vi "Sub_TaD.vi"() -> ()   [LabVIEW 2020]
panel:
  out "Actual\ntime":string
  in  "STOP":bool
  in  "DATE":bool
  in  "YEAR":i32=2020 min=2010 max=2070 step=1
  in  "MONTH":i32=6 min=1 max=12 step=1
  in  "DAY":i32=15 min=1 max=31 step=1
  in  "TIME":bool
  in  "MINUTE":i32=30 min=-1 max=60 step=1
  in  "HOUR":i32=12 min=-1 max=24 step=1
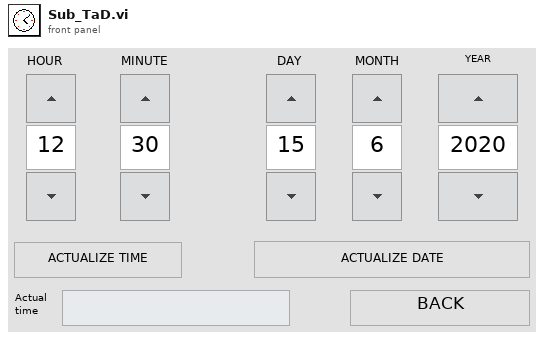
[diagram p1: front panel]
types:
  T1 = enum16{"open", "replace", "create", "open or create", "replace or create", "replace or create with confirmation"}
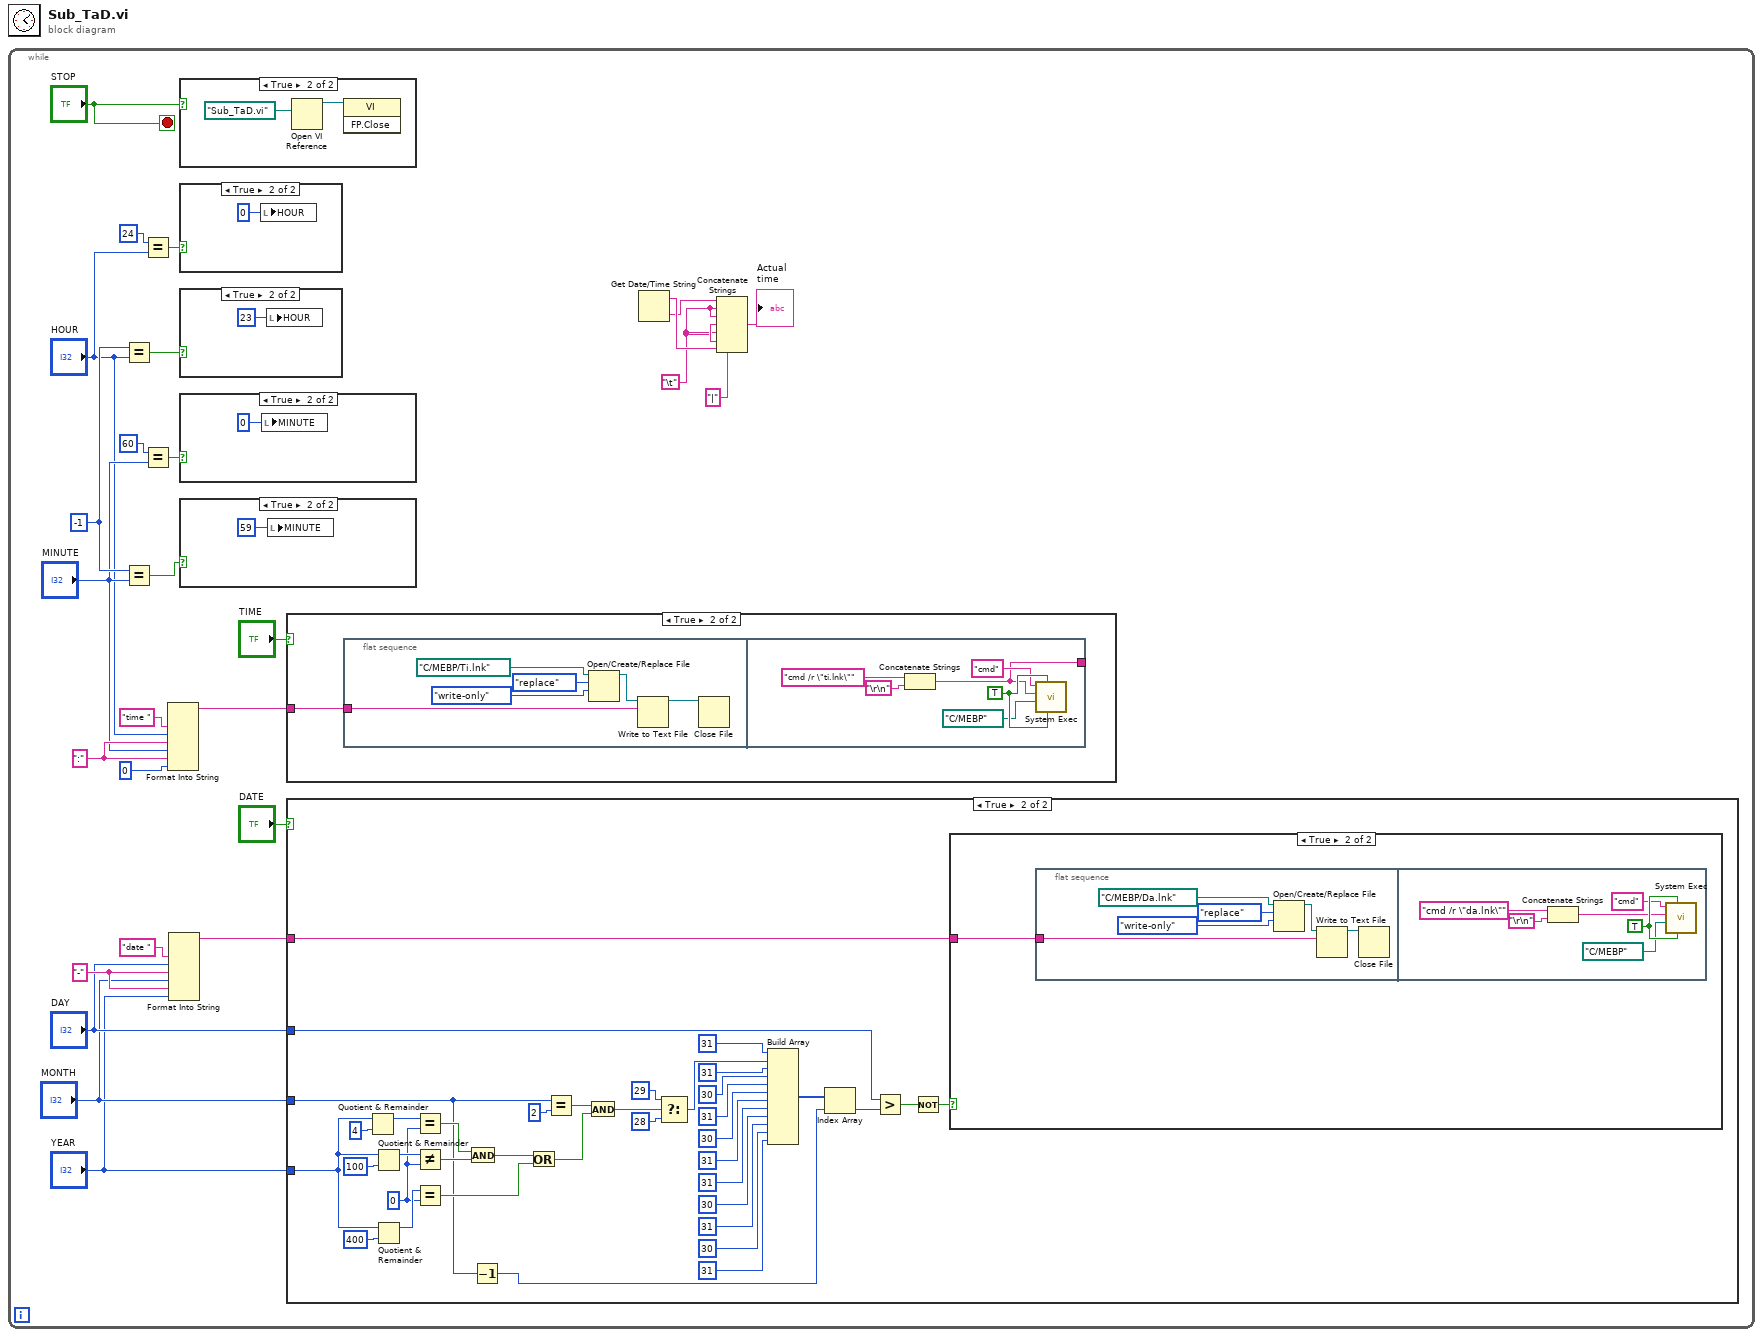
[diagram p0: block diagram]
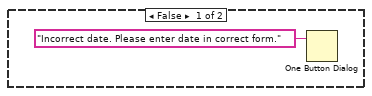
[diagram p4: hidden frame]
diagram:
  n1 = while {
    stop <- "STOP" stop-if-true
    w2 = "\t"
    w13 = "-"
    w24 = -1
    w26 = ":"
    n2 = Equal?(x=w24, y="HOUR") -> (x = y?=w20:bool)
    n3 = Equal?(x=w24, y="MINUTE") -> (x = y?=w19:bool)
    n4 = Equal?(x=24, y="HOUR") -> (x = y?=w21:bool)
    n5 = Equal?(x=60, y="MINUTE") -> (x = y?=w18:bool)
    n6 = Format Into String("time " ("string"), "HOUR", w26, "MINUTE", w26, 0 ("input 6")) -> (resulting string=w11:string)  [unwired: 3 in, 1 out]
    n7 = Format Into String("date " ("string"), "DAY", w13, "MONTH", w13, "YEAR") -> (resulting string=w10:string)  [unwired: 3 in, 1 out]
    n8 = case shown="True" "STOP" {
      frame False {
      }
      frame True {
        n9 = Open VI Reference(vi path=path "Sub_TaD.vi") -> (vi reference=w28:refnum<vi>)  [unwired: 5 in, 1 out]
        n10 = invoke class="VI" method="FP.Close"(reference=w28) -> ()  [unwired: 2 in, 3 out]
      }
    }
    n11 = case shown="True" w21 {
      frame False {
      }
      frame True {
        n12 = local write "HOUR"(0 ("Numeric")) -> ()
      }
    }
    n13 = case shown="True" w20 {
      frame False {
      }
      frame True {
        n14 = local write "HOUR"(23 ("Numeric")) -> ()
      }
    }
    n15 = case shown="True" w18 {
      frame False {
      }
      frame True {
        n16 = local write "MINUTE"(0 ("Numeric 2")) -> ()
      }
    }
    n17 = case shown="True" w19 {
      frame False {
      }
      frame True {
        n18 = local write "MINUTE"(59 ("Numeric 2")) -> ()
      }
    }
    n19 = case shown="True" "TIME" {
      tunnel: w11 -> [_ w82]
      frame False {
      }
      frame True {
        n20 = flat-sequence {
          tunnel: w82 -> [w83]
          tunnel: [w89] -> _
          frame #0 {
            n21 = Open/Create/Replace File(file path (use dialog)=path "C:/MEBP/Ti.lnk", operation (0:open)=T1."replace", access (0:read/write)=enum16{"read/write", "read-only", "write-only"}."write-only") -> (refnum out=w87:refnum<file>)  [unwired: 3 in, 2 out]
            n22 = Write to Text File(file (use dialog)=w87, text=w83) -> (refnum out=w88:refnum<file>)  [unwired: 2 in, 2 out]
            n23 = Close File(refnum=w88) -> ()  [unwired: 1 in, 2 out]
          }
          frame #1 {
            w94 = TRUE ("wait until completion? (T)")
            n24 = Concatenate Strings("cmd /r \"ti.lnk\"", "\r\n") -> (w89:string)
            n25 = call <vilib>:"System Exec.vi"("run minimized? (F)"=w94, "wait until completion? (T)"=w94, "working directory"=path "C:/MEBP", "standard input"=w89, "command line"="cmd") -> ()  [unwired: 3 in, 4 out]
          }
        }
      }
    }
    n26 = case shown="True" "DATE" {
      tunnel: w10 -> [_ w53]
      tunnel: "DAY" -> [_ w65]
      tunnel: "MONTH" -> [_ w31]
      tunnel: "YEAR" -> [_ w47]
      frame False {
      }
      frame True {
        w41 = 0 ("y")
        n27 = Quotient & Remainder(x=w47, y=4) -> (x-y*floor(x/y)=w50:i32)  [unwired: 1 out]
        n28 = Quotient & Remainder(x=w47, y=100) -> (x-y*floor(x/y)=w45:i32)  [unwired: 1 out]
        n29 = Quotient & Remainder(x=w47, y=400) -> (x-y*floor(x/y)=w42:i32)  [unwired: 1 out]
        n30 = Equal?(x=w50, y=w41) -> (x = y?=w43:bool)
        n31 = Not Equal?(x=w45, y=w41) -> (x != y?=w44:bool)
        n32 = Equal?(x=w42, y=w41) -> (x = y?=w39:bool)
        n33 = And(x=w43, y=w44) -> (x .and. y?=w40:bool)
        n34 = Decrement(x=w31) -> (x-1=w30:i32)
        n35 = Or(x=w40, y=w39) -> (x .or. y?=w37:bool)
        n36 = Equal?(x=w31, y=2) -> (x = y?=w38:bool)
        n37 = And(x=w38, y=w37) -> (x .and. y?=w36:bool)
        n38 = Select(t=29, s=w36, f=28) -> (s? t:f=w33:i32)
        n39 = Build Array(31, w33, 31, 30, 31, 30, 31, 31, 30, 31, 30, 31) -> (w66:i32[])
        n40 = Index Array(array=w66, index=w30) -> (element=w67:i32)
        n41 = Greater?(x=w65, y=w67) -> (0:w52:bool)
        n42 = Not(x=w52) -> (.not. x?=w32:bool)
        n43 = case shown="True" w32 {
          tunnel: w53 -> [_ w69]
          frame False {
            n44 = One Button Dialog(message="Incorrect date. Please enter date in correct form.") -> ()  [unwired: 1 in, 1 out]
          }
          frame True {
            n45 = flat-sequence {
              tunnel: w69 -> [w70]
              frame #0 {
                n46 = Open/Create/Replace File(file path (use dialog)=path "C:/MEBP/Da.lnk", operation (0:open)=T1."replace", access (0:read/write)=enum16{"read/write", "read-only", "write-only"}."write-only") -> (refnum out=w74:refnum<file>)  [unwired: 3 in, 2 out]
                n47 = Write to Text File(file (use dialog)=w74, text=w70) -> (refnum out=w75:refnum<file>)  [unwired: 2 in, 2 out]
                n48 = Close File(refnum=w75) -> ()  [unwired: 1 in, 2 out]
              }
              frame #1 {
                w81 = TRUE ("wait until completion? (T)")
                n49 = Concatenate Strings("cmd /r \"da.lnk\"", "\r\n") -> (w76:string)
                n50 = call <vilib>:"System Exec.vi"("run minimized? (F)"=w81, "wait until completion? (T)"=w81, "working directory"=path "C:/MEBP", "standard input"=w76, "command line"="cmd") -> ()  [unwired: 3 in, 4 out]
              }
            }
          }
        }
      }
    }
    n51 = Get Date/Time String() -> (date string=w4:string, time string=w3:string)  [unwired: 3 in]
    n52 = Concatenate Strings(w3, w2, w2, "|", w2, w2, w4) -> (→"Actual\ntime":string)
  }
